vi "属性节点.vi"() -> ()   [LabVIEW 2018]
panel:
  in  "游标":dbl(slide) min=0.0 max=1.0 scale=0.0..1.0
  in  "Y轴平移":dbl(knob) min=-5.0 max=5.0 scale=-5.0..5.0
  in  "Y轴缩放":dbl(knob) min=0.0 max=5.0 scale=0.0..5.0
  in  "X轴平移":dbl(knob) min=-5.0 max=5.0 scale=-5.0..5.0
  in  "自动调整":bool
  in  "停止":bool
  in  "X轴缩放":dbl(knob) scale=0.0..10.0
  out "波形图":dynamicdata(graph)
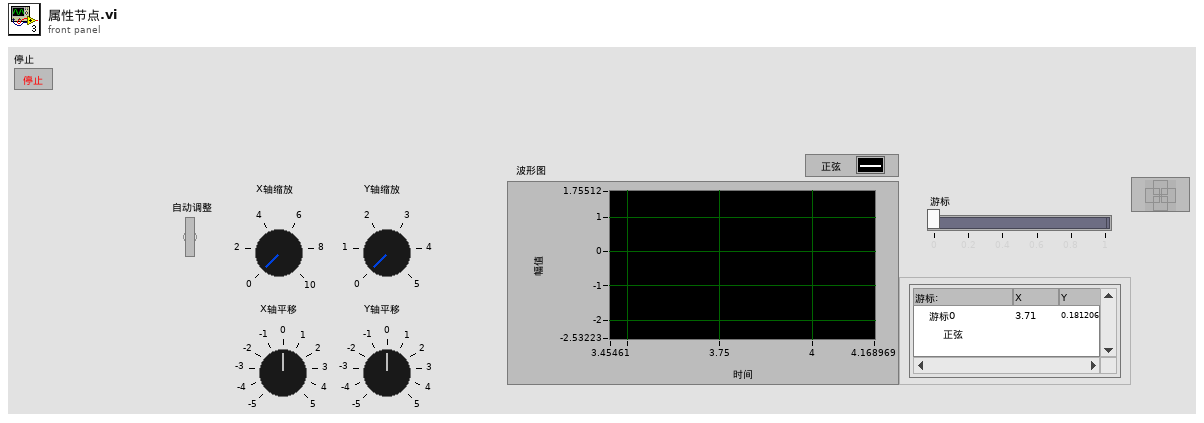
[diagram p1: front panel]
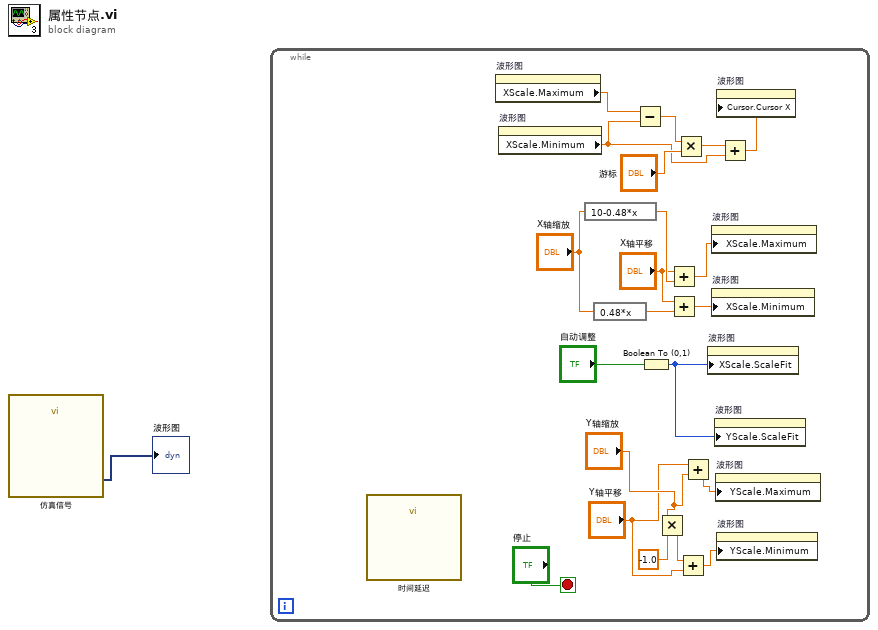
[diagram p0: block diagram]
diagram:
  n1 = call "仿真信号"() -> ("正弦"=→"波形图":dynamicdata)  [unwired: 14 in, 1 out]
  n2 = while {
    stop <- "停止" stop-if-true
    n3 = call "时间延迟"() -> ()  [unwired: 11 in, 1 out]
    n4 = property on="波形图" class="WFGraph (严格)"() -> ("XScale.Maximum"=w7:dbl)  [unwired: 2 in, 2 out]
    n5 = property on="波形图" class="WFGraph (严格)"() -> ("XScale.Minimum"=w3:dbl)  [unwired: 2 in, 2 out]
    n6 = expression code="10-0.48*x"("X轴缩放") -> (w18:dbl)
    n7 = expression code="0.48*x"("X轴缩放") -> (w20:dbl)
    n8 = Subtract(x=w7, y=w3) -> (x-y=w6:dbl)
    n9 = Boolean To (0,1)(Boolean="自动调整") -> (0, 1=w15:i16)
    n10 = Multiply(x="Y轴缩放", y=-1.0) -> (x*y=w12:dbl)
    n11 = Add(x="X轴平移", y=w18) -> (x+y=w16:dbl)
    n12 = Add(x="X轴平移", y=w20) -> (x+y=w19:dbl)
    n13 = Multiply(x=w6, y="游标") -> (x*y=w4:dbl)
    n14 = Add(x=w12, y="Y轴平移") -> (x+y=w11:dbl)
    n15 = Add(x="Y轴平移", y="Y轴缩放") -> (x+y=w13:dbl)
    n16 = property on="波形图" class="WFGraph (严格)"("XScale.ScaleFit"=w15) -> ()  [unwired: 2 in, 2 out]
    n17 = property on="波形图" class="WFGraph (严格)"("XScale.Maximum"=w16) -> ()  [unwired: 2 in, 2 out]
    n18 = property on="波形图" class="WFGraph (严格)"("XScale.Minimum"=w19) -> ()  [unwired: 2 in, 2 out]
    n19 = property on="波形图" class="WFGraph (严格)"("YScale.ScaleFit"=w15) -> ()  [unwired: 2 in, 2 out]
    n20 = property on="波形图" class="WFGraph (严格)"("YScale.Maximum"=w13) -> ()  [unwired: 2 in, 2 out]
    n21 = property on="波形图" class="WFGraph (严格)"("YScale.Minimum"=w11) -> ()  [unwired: 2 in, 2 out]
    n22 = Add(x=w4, y=w3) -> (x+y=w2:dbl)
    n23 = property on="波形图" class="WFGraph (严格)"("Cursor.Cursor X"=w2) -> ()  [unwired: 2 in, 2 out]
  }
